vi "Get Async FIFO Refs.vi"(8 "error in":errorcluster, 10 "Data Access API In":refnum<class "Data Access Engine.lvclass">, 11 "Async State Vars In":T1) -> (0 "error out":errorcluster, 2 "Data Access API Out":refnum<class "Data Access Engine.lvclass">, 3 "Async State Vars Out":T1)   [LabVIEW 2017, in "Waveform-Processing-Custom-Device Engine.lvlib"]
uses:
  Waveform-Processing-Custom-Device Engine.lvlib
  Types/AsyncStateVariables.ctl
  <vilib>/NI VeriStand/Custom Device Waveform API/Single Waveform Read (DBL)/Single Waveform Read (DBL).lvclass
  <vilib>/NI VeriStand/Custom Device Waveform API/Single Waveform Write (DBL)/Single Waveform Write (DBL).lvclass
  <vilib>/NI Veristand/Custom Device API/Waveform Data Reference.ctl
  Types/New Async FIFOs.ctl
  <vilib>/NI/NIVS Inline Async API/_Data Access Engine/Data Access Engine/Types/Write.DVR.ctl
  <vilib>/NI/NIVS Inline Async API/_Data Access Engine/Access Type Classes/Write/Write.lvclass
  <vilib>/NI/NIVS Inline Async API/_Data Access Engine/Data Access Engine/Data Access Engine.lvclass
  Shared/Constants.vi
  <vilib>/NI/NIVS Inline Async API/_Data Access Engine/Data Access Engine/Methods/Write.Lookup.vi
  Shared/Waveform-Processing-Custom-Device Shared.lvlib
  <vilib>/NI Veristand/Custom Device API/Custom Device API.lvlib
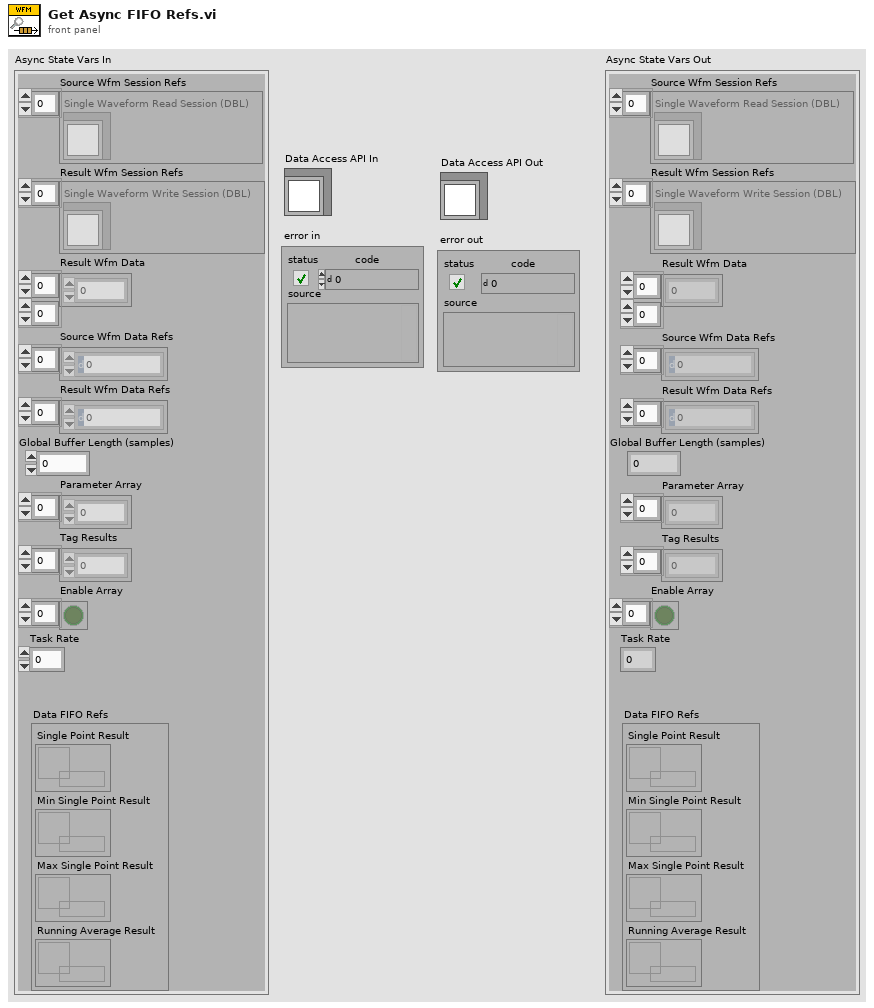
[diagram p1: front panel]
types:
  T1 = typedef "Waveform-Processing-Custom-Device Engine.lvlib/AsyncStateVariables.ctl" = cluster{"Source Wfm Session Refs":refnum<class "Single Waveform Read (DBL).lvclass">[], "Result Wfm Session Refs":refnum<class "Single Waveform Write (DBL).lvclass">[], "Result Wfm Data":dbl[][], "Source Wfm Data Refs":T2[], "Result Wfm Data Refs":T2[], "Global Buffer Length (samples)":dbl, "Parameter Array":dbl[], "Tag Results":dbl[], "Enable Array":bool[], "Task Rate":dbl, "Data FIFO Refs":T3}
  T2 = typedef "Custom Device API.lvlib/Waveform Data Reference.ctl" = i32
  T3 = typedef "Waveform-Processing-Custom-Device Engine.lvlib/New Async FIFOs.ctl" = cluster{"Single Point Result":T4, "Running Average Result":T4, "Min Single Point Result":T4, "Max Single Point Result ":T4}
  T4 = typedef "Data Access Engine.lvlib/Data Access Engine.lvclass/Write.DVR.ctl" = refnum<data-value>
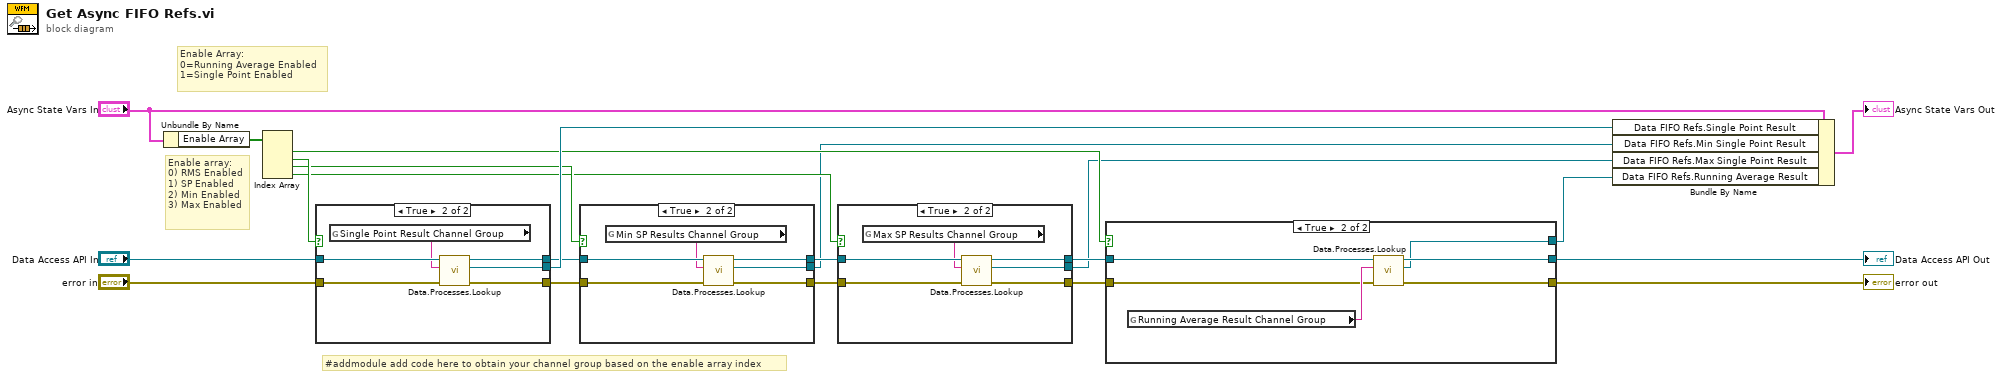
[diagram p0: block diagram]
diagram:
  # "Enable array:\n0) RMS Enabled\n1) SP Enabled\n2) Min Enabled\n3) Max Enabled"
  # "#addmodule add code here to obtain your channel group based on the enable array index"
  # "Enable Array:\n0=Running Average Enabled\n1=Single Point Enabled"
  n1 = Unbundle By Name("Async State Vars In") -> ("Enable Array"=w14:bool[])
  n2 = Index Array(array=w14) -> (element #1=w12:bool, element #2=w13:bool, element #3=w9:bool, element #4=w6:bool)  [unwired: 4 in]
  n3 = case shown="True" w13 {
    tunnel: "Data Access API In" -> [w23 w29]
    tunnel: [w23 w28] -> w11
    tunnel: "error in" -> [w22 w27]
    tunnel: [_ w26] -> w17
    tunnel: [w22 w24] -> w10
    frame False {
      # "If single point is not enabled, \npass data through and create \ndefault refnum for FIFO"
    }
    frame True {
      n4 = global read "Constants.vi" "Single Point Result Channel Group"() -> (w25:string)
      n5 = call-poly <vilib>:"Data.Processes.Lookup.vi"("error in (no error)"=w27, "Name"=w25, "Data Access API in"=w29) -> ("error out"=w24:errorcluster, "Ref"=w26:T4, "Data Access API out"=w28:refnum<class "Data Access Engine.lvclass">)  [unwired: 5 in, 1 out]
    }
  }
  n6 = case shown="True" w9 {
    tunnel: w11 -> [w31 w37]
    tunnel: [w31 w36] -> w8
    tunnel: w10 -> [w30 w35]
    tunnel: [_ w34] -> w2
    tunnel: [w30 w33] -> w7
    frame False {
      # "If Min single point is not enabled, \npass data through and create \ndefault refnum for FIFO"
    }
    frame True {
      n7 = global read "Constants.vi" "Min SP Results Channel Group"() -> (w32:string)
      n8 = call-poly <vilib>:"Data.Processes.Lookup.vi"("error in (no error)"=w35, "Name"=w32, "Data Access API in"=w37) -> ("error out"=w33:errorcluster, "Ref"=w34:T4, "Data Access API out"=w36:refnum<class "Data Access Engine.lvclass">)  [unwired: 5 in, 1 out]
    }
  }
  n9 = case shown="True" w6 {
    tunnel: w8 -> [w39 w45]
    tunnel: [w39 w44] -> w5
    tunnel: w7 -> [w38 w43]
    tunnel: [_ w42] -> w1
    tunnel: [w38 w41] -> w4
    frame False {
      # "If Min single point is not enabled, \npass data through and create \ndefault refnum for FIFO"
    }
    frame True {
      n10 = global read "Constants.vi" "Max SP Results Channel Group"() -> (w40:string)
      n11 = call-poly <vilib>:"Data.Processes.Lookup.vi"("error in (no error)"=w43, "Name"=w40, "Data Access API in"=w45) -> ("error out"=w41:errorcluster, "Ref"=w42:T4, "Data Access API out"=w44:refnum<class "Data Access Engine.lvclass">)  [unwired: 5 in, 1 out]
    }
  }
  n12 = case shown="True" w12 {
    tunnel: [w46 w53] -> w21
    tunnel: w5 -> [w46 w52]
    tunnel: [w47 w50] -> w16
    tunnel: w4 -> [w47 w49]
    tunnel: [_ w48] -> w3
    frame False {
      # "If running average is not enabled, pass data through\nand create default refnum for both FIFOs"
    }
    frame True {
      n13 = global read "Constants.vi" "Running Average Result Channel Group"() -> (w51:string)
      n14 = call-poly <vilib>:"Data.Processes.Lookup.vi"("error in (no error)"=w49, "Name"=w51, "Data Access API in"=w52) -> ("error out"=w50:errorcluster, "Ref"=w48:T4, "Data Access API out"=w53:refnum<class "Data Access Engine.lvclass">)  [unwired: 5 in, 1 out]
    }
  }
  "error out" <- w16
  "Data Access API Out" <- w21
  n15 = Bundle By Name(cluster="Async State Vars In", "Data FIFO Refs.Single Point Result"=w17, "Data FIFO Refs.Min Single Point Result"=w2, "Data FIFO Refs.Max Single Point Result"=w1, "Data FIFO Refs.Running Average Result"=w3) -> (→"Async State Vars Out":T1)
